vi "Calculate Vision Target Angle.vi"(9 "Target Distance (ft)":dbl, 11 "Target Width (cam Pct)":dbl) -> (2 "Target Angle":dbl)   [LabVIEW 2013]
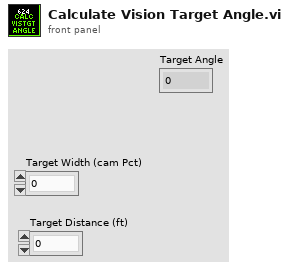
[diagram p1: front panel]
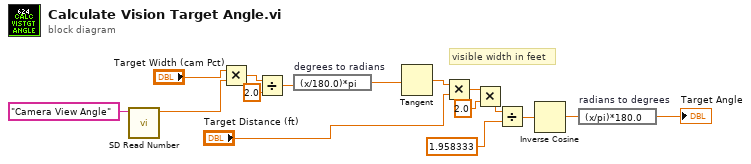
[diagram p0: block diagram]
diagram:
  # "visible width in feet"
  n1 = call <vilib>:"SD Read Number.vi"("Name"="Camera View Angle") -> ("Numeric"=w4:dbl)  [unwired: 8 in, 2 out]
  n2 = Multiply(x="Target Width (cam Pct)", y=w4) -> (x*y=w2:dbl)
  n3 = Divide(x=w2, y=2.0) -> (x/y=w3:dbl)
  n4 = expression code="(x/180.0)*pi" "degrees to radians"(w3) -> (w16:dbl)
  n5 = Tangent(1:w16) -> (0:w15:dbl)
  n6 = Multiply(x=w15, y="Target Distance (ft)") -> (x*y=w11:dbl)
  n7 = Multiply(x=w11, y=2.0) -> (x*y=w9:dbl)
  n8 = Divide(x=w9, y=1.958333) -> (x/y=w13:dbl)
  n9 = Inverse Cosine(1:w13) -> (0:w8:dbl)
  n10 = expression code="(x/pi)*180.0" "radians to degrees"(w8) -> (→"Target Angle":dbl)
